vi "Read Device Fault.vi"(0 "reference in":refnum<class "Power Supply.lvclass">, 5 "error in (no error)":errorcluster) -> (14 "reference out":refnum<class "Power Supply.lvclass">, 16 "Power Supply Error":bool, 17 "Fault Register":u8, 19 "error out":errorcluster)   [LabVIEW 2017, in "Power Supply.lvclass"]
uses:
  Power Supply.lvclass
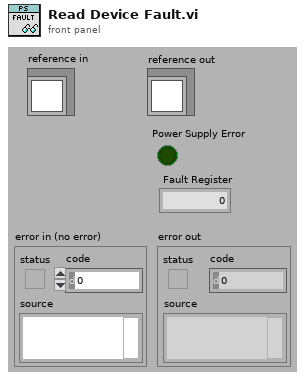
[diagram p1: front panel]
types:
  T1 = typedef "Power Supply.lvclass/ObjectAttributes.ctl" = cluster{"Power Supply Chain VISA Session":refnum<visa-resource-name>, "Power Supply Chain Address":i16, "Power Supply Open/Close Status":bool, "Power Supply Voltage Setting":dbl, "Power Supply Current Setting":dbl, "Power Supply Voltage Reading":dbl, "Power Supply Current Reading":dbl, "Power Supply Status":T2, "Power Supply Error":T3, "Fault Register":u8, "Power Supply Error":bool}
  T2 = typedef "Power Supply.lvclass/Power Supply Status.ctl" = enum16{"Closed", "Open"}
  T3 = typedef "Power Supply.lvclass/Power Supply Error.ctl" = enum16{"None", "Read Error"}
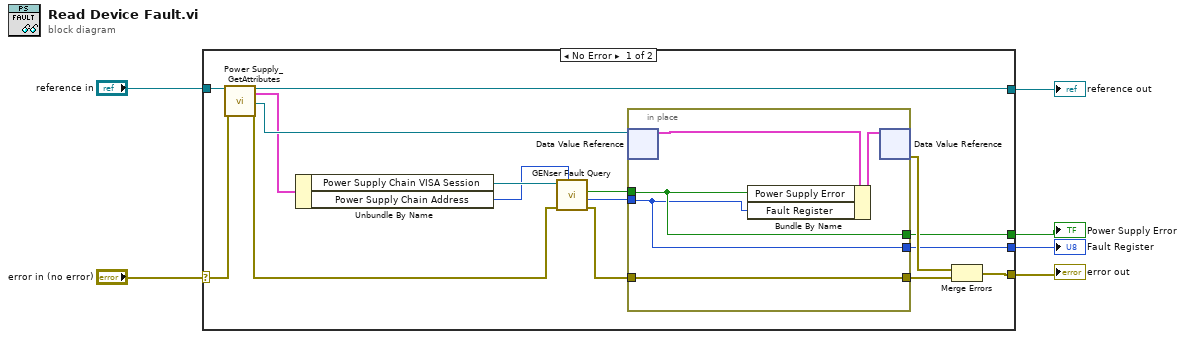
[diagram p0: block diagram]
diagram:
  n1 = case shown="No Error" "error in (no error)" {
    selector: "error in (no error)" -> [w21 w29]
    tunnel: [w18 w29] -> w5
    tunnel: [w19 w28] -> w3
    tunnel: "reference in" -> [w22 w28]
    tunnel: [w15 _] -> w2
    tunnel: [w14 _] -> w1
    frame No Error {
      n2 = call "Power Supply_GetAttributes.vi"("reference in"=w22, "error in (no error)"=w21) -> ("reference out"=w19:refnum<class "Power Supply.lvclass">, "Data"=w11:T1, "DataRef"=w17:refnum<data-value>, "error out"=w8:errorcluster)  [unwired: 14 in]
      n3 = Unbundle By Name(w11) -> ("Power Supply Chain VISA Session"=w13:refnum<visa-resource-name>, "Power Supply Chain Address"=w12:i16)
      n4 = call <instrlib>:"GENser Fault Query.vi"("GEN Addr"=w12, "error"=w8, "VISA"=w13) -> ("error out"=w7:errorcluster, "Fault Register"=w9:u8, "Fault?"=w10:bool)  [unwired: 4 in, 2 out]
      n5 = in-place {
        in-place-border: w7 -> [w23]
        in-place-border: [w23] -> w16
        in-place-border: [w24] -> w15
        in-place-border: [w25] -> w14
        in-place-border: w10 -> [w25]
        in-place-border: w9 -> [w24]
        n6 = in-place-dvr #1(w17) -> (w26:T1)  [unwired: 1 out]
        n7 = Bundle By Name(cluster=w26, "Power Supply Error"=w25, "Fault Register"=w24) -> (w27:T1)
        n8 = in-place-dvr #1(w27) -> (w20:errorcluster)  [unwired: 1 out]
      }
      n9 = Merge Errors(w20, w16) -> (w18:errorcluster)
    }
    frame Error {
    }
  }
  "error out" <- w5
  "reference out" <- w3
  "Power Supply Error" <- w1
  "Fault Register" <- w2
